vi "SetSettings.vi"(8 "Error In":errorcluster[](array[cluster]), 10 "XmlData":string) -> (0 "Error Out":errorcluster[](array[cluster]))   [LabVIEW 2017, in "Bus_class.lvlib" / "Bus.lvclass"]
uses:
  Bus.lvclass
  Config_class/Config.lvclass/Config.ctl
  Config_class/Read Logging.vi
  Config_class/Accessors/Read PARTF Root Directory.vi
  Config_class/Accessors/Write PARTF Root Directory.vi
  Config_class/Accessors/Write ConfigFilePath.vi
  Config_class/Accessors/Write Logging.vi
  Config_class/Config.lvclass
  <userlib>/NIST/NISTErrorLib/NISTErrorLib.lvlib
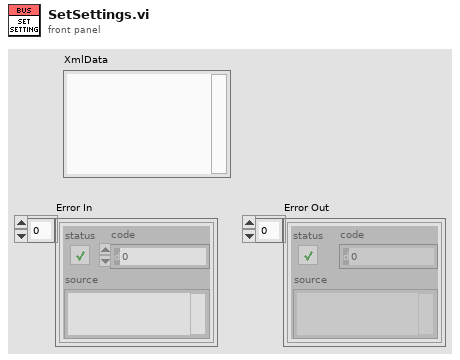
[diagram p1: front panel]
types:
  T1 = cluster{"RootDir":string, "TestDir":string, "ScriptDir":string, "OutDir":string, "ConfigFilePath":string, "Log File Path":string}
  T2 = typedef "Framework.lvlib/Config.lvclass/Logging.ctl" = cluster{"eLogLvl":T3, "Log File Path":path, "btnLogFile":bool}
  T3 = typedef "Framework.lvlib/Config.lvclass/eLogLvl.ctl" = enum16{"Normal", "Verbose", "None"}
  T4 = typedef "Framework.lvlib/Config.lvclass/RootDir.ctl" = cluster{"pathRootDir":path, "btnOutPath":bool, "OutDir":string, "btnOpenOutputDir":bool, "ScriptDir":string, "btnOpenScriptDir":bool, "TestDir":string, "btnOpenTestDir":bool}
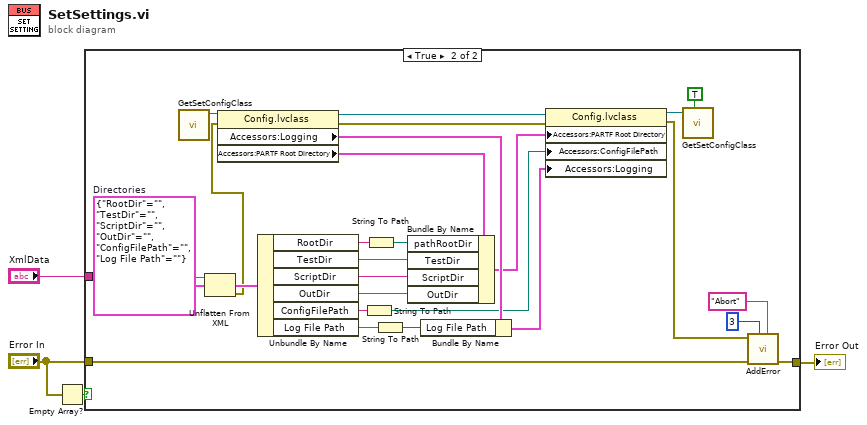
[diagram p0: block diagram]
diagram:
  n1 = Empty Array?(array="Error In") -> (empty?=w4:bool)
  n2 = case shown="True" w4 {
    tunnel: [w5 w12] -> w2
    tunnel: "Error In" -> [w5 w13]
    tunnel: "XmlData" -> [_ w28]
    frame False {
    }
    frame True {
      w29 = T1 {"RootDir"="", "TestDir"="", "ScriptDir"="", "OutDir"="", "ConfigFilePath"="", "Log File Path"=""}  # Directories
      n3 = call "GetSetConfigClass.vi"() -> ("Ref out"=w32:refnum<class "Config.lvclass">)  [unwired: 11 in]
      n4 = Unflatten From XML(xml string=w28, type=w29) -> (value=w30:T1, error out=w15:errorcluster)  [unwired: 1 in]
      n5 = property class="Config.lvclass"(reference=w32, error in=w15) -> (reference out=w22:refnum<class "Config.lvclass">, error out=w14:errorcluster, "Accessors:Logging"=w20:T2, "Accessors:PARTF Root Directory"=w21:T4)
      n6 = Unbundle By Name(w30) -> ("RootDir"=w26:string, "TestDir"=w25:string, "ScriptDir"=w24:string, "OutDir"=w23:string, "ConfigFilePath"=w18:string, "Log File Path"=w27:string)
      n7 = String To Path(string=w18) -> (path=w7:path)
      n8 = String To Path(string=w26) -> (path=w8:path)
      n9 = String To Path(string=w27) -> (path=w6:path)
      n10 = Bundle By Name(cluster=w21, "pathRootDir"=w8, "TestDir"=w25, "ScriptDir"=w24, "OutDir"=w23) -> (w19:T4)
      n11 = Bundle By Name(cluster=w20, "Log File Path"=w6) -> (w17:T2)
      n12 = property class="Config.lvclass"(reference=w22, error in=w14, "Accessors:PARTF Root Directory"=w19, "Accessors:ConfigFilePath"=w7, "Accessors:Logging"=w17) -> (reference out=w16:refnum<class "Config.lvclass">, error out=w11:errorcluster)
      n13 = call "GetSetConfigClass.vi"("Set (f)"=TRUE, "Ref in"=w16) -> ()  [unwired: 9 in, 1 out]
      n14 = call <userlib>:"AddError.vi"("Severity"="Abort", "Priority"=u8 3, "ErrorArray"=w13, "error in (no error)"=w11) -> ("ErrorArray"=w12:errorcluster[])  [unwired: 6 in, 1 out]
    }
  }
  "Error Out" <- w2
